vi "receiveData.vi"(8 "error in (no error)":errorcluster, 11 "Model in":refnum<class "Model.lvclass">) -> (0 "error out":errorcluster, 3 "Model out":refnum<class "Model.lvclass">)   [LabVIEW 2015, in "Model.lvclass"]
uses:
  Model.lvclass
  Typedefs/InputData.ctl
  Typedefs/ForceDemand.ctl
  <userlib>/Common/Devices/DistanceGauge/Typedefs/Distance Data.ctl
  Model.lvclass/Model.ctl
  UserEvents/UserEvents.lvclass/UserEvents.ctl
  <userlib>/Common/Devices/DistanceGauge/DistanceGauge/DistanceGauge.lvclass/DistanceGauge.ctl
  <userlib>/Common/ILC/ILC/ILC.lvclass/ILC.ctl
  <userlib>/Common/Devices/ForceSensorCalculator/ForceSensorCalculator/ForceSensorCalculator.lvclass/ForceSensorCalculator.ctl
  ApplicationElements/Log/TestDataLog/TestDataLog.lvclass/TestDataLog.ctl
  <userlib>/Common/ILC/ILC/ILC.lvclass
  <userlib>/Common/Devices/DistanceGauge/DistanceGauge/DistanceGauge.lvclass
  <userlib>/Common/Devices/ForceSensorCalculator/ForceSensorCalculator/ForceSensorCalculator.lvclass
  Typedefs/M1M3SSSTypedefs.lvlib
  <userlib>/Common/Devices/DistanceGauge/DistanceGauge.lvlib
  UserEvents/UserEvents.lvclass
  ApplicationElements/Log/TestDataLog/TestDataLog.lvclass
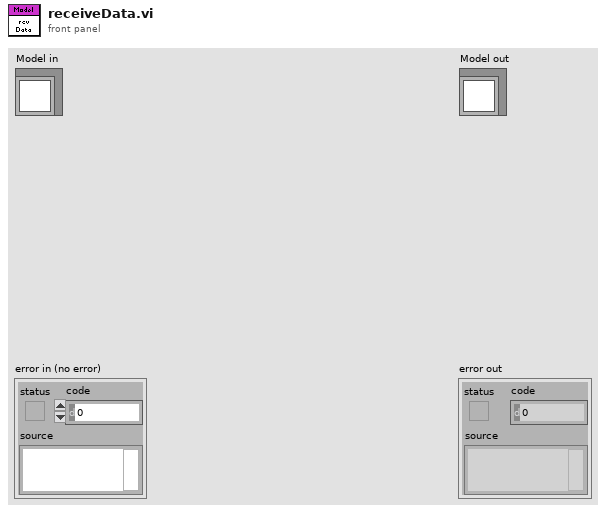
[diagram p1: front panel]
types:
  T1 = typedef "M1M3SSSTypedefs.lvlib/InputData.ctl" = cluster{"Force Measured":T2, "Distance Data":T3}
  T2 = typedef "M1M3SSSTypedefs.lvlib/ForceDemand.ctl" = dbl[unit]
  T3 = typedef "DistanceGauge.lvlib/Distance Data.ctl" = cluster{"Distance Measured 1":dbl[unit], "Distance Measured 2":dbl[unit]}
  T4 = typedef "M1M3SSSTypedefs.lvlib/PubDataEvents.ctl" = cluster{"State":refnum<user-event>, "ErrorCode":refnum<user-event>, "OutputData":refnum<user-event>, "InputData":refnum<user-event>, "ControllerData":refnum<user-event>, "TestStatus":refnum<user-event>, "LogPath":refnum<user-event>, "StiffnessData":refnum<user-event>, "PreconditioningCycle":refnum<user-event>}
  T5 = typedef "ILCCommon.lvlib/ILCTypedefs.lvlib/ADCsInEngineeringUnits.ctl" = cluster{"Ch1":dbl[unit], "Ch2":dbl[unit], "Ch3":dbl[unit], "Ch4":dbl[unit]}
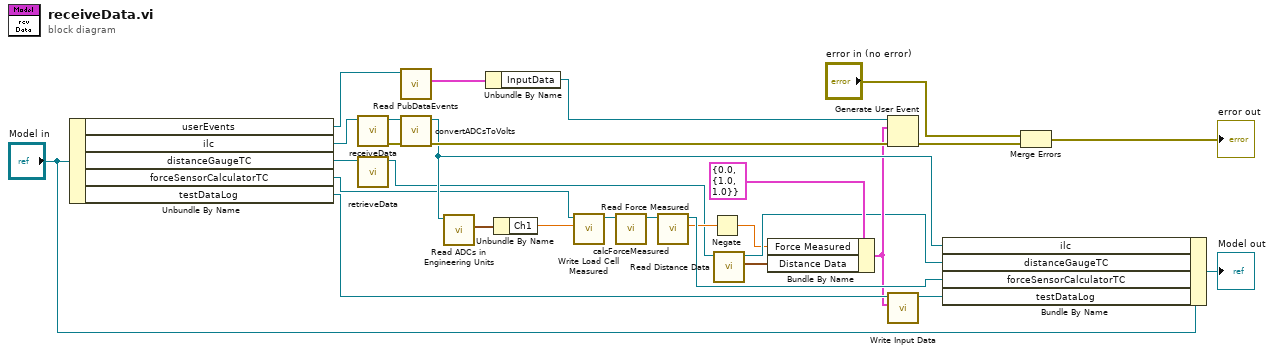
[diagram p0: block diagram]
diagram:
  n1 = Unbundle By Name("Model in") -> ("userEvents"=w13:refnum<class "UserEvents.lvclass">, "ilc"=w8:refnum<class "ILC.lvclass">, "distanceGaugeTC"=w27:refnum<class "DistanceGaugeTC.lvclass">, "forceSensorCalculatorTC"=w5:refnum<class "ForceSensorCalculatorTC.lvclass">, "testDataLog"=w16:refnum<class "TestDataLog.lvclass">)
  n2 = call <userlib>:"receiveData.vi"("ILC in"=w8) -> ("error out"=w22:errorcluster, "ILC out"=w23:refnum<class "ILC.lvclass">)  [unwired: 9 in]
  n3 = call <userlib>:"retrieveData.vi"("DistanceGauge in"=w27) -> ("DistanceGauge out"=w4:refnum<class "DistanceGaugeTC.lvclass">)  [unwired: 8 in, 2 out]
  n4 = call "Read PubDataEvents.vi"("UserEvents in"=w13) -> ("PubDataEvents"=w9:T4)  [unwired: 9 in, 1 out]
  n5 = call <userlib>:"convertADCsToVolts.vi"("error in (no error)"=w22, "ILC in"=w23) -> ("error out"=w21:errorcluster, "ILC out"=w12:refnum<class "ILC.lvclass">)  [unwired: 8 in]
  n6 = call <userlib>:"Read ADCs in Engineering Units.vi"("ILC in"=w12) -> ("ADCs in Engineering Units"=w20:T5)  [unwired: 9 in, 1 out]
  n7 = Unbundle By Name(w9) -> ("InputData"=w14:refnum<user-event>)
  n8 = Unbundle By Name(w20) -> ("Ch1"=w7:dbl[unit])
  n9 = call <userlib>:"Write Load Cell Measured.vi"("Load Cell Measured"=w7, "ForceSensor in"=w5) -> ("ForceSensor out"=w6:refnum<class "ForceSensorCalculatorTC.lvclass">)  [unwired: 9 in]
  n10 = call <userlib>:"calcForceMeasured.vi"("ForceSensor in"=w6) -> ("ForceSensor out"=w19:refnum<class "ForceSensorCalculatorTC.lvclass">)  [unwired: 9 in, 1 out]
  n11 = call <userlib>:"Read Force Measured.vi"("ForceSensor in"=w19) -> ("Force Demand"=w10:dbl[unit], "ForceSensor out"=w18:refnum<class "ForceSensorCalculatorTC.lvclass">)  [unwired: 9 in]
  n12 = Negate(x=w10) -> (-x=w1:dbl[unit])
  n13 = call <userlib>:"Read Distance Data.vi"("DistanceGauge in"=w4) -> ("Distance Data"=w2:T3, "DistanceGauge out"=w3:refnum<class "DistanceGaugeTC.lvclass">)  [unwired: 9 in]
  n14 = Bundle By Name(cluster=T1 {"Force Measured"=0.0, "Distance Data"={"Distance Measured 1"=1.0, "Distance Measured 2"=1.0}} ("event data"), "Force Measured"=w1, "Distance Data"=w2) -> (w11:T1)
  n15 = Generate User Event(user event=w14, event data cluster=w11, error in=w21) -> (error out=w25:errorcluster)  [unwired: 1 in, 1 out]
  n16 = call "Write Input Data.vi"("Input Data"=w11, "Logger in"=w16) -> ("Logger out"=w15:refnum<class "TestDataLog.lvclass">)  [unwired: 9 in]
  n17 = Bundle By Name(cluster="Model in", "ilc"=w12, "distanceGaugeTC"=w3, "forceSensorCalculatorTC"=w18, "testDataLog"=w15) -> (→"Model out":refnum<class "Model.lvclass">)
  n18 = Merge Errors("error in (no error)", w25) -> (→"error out":errorcluster)
